vi "Control Panel.vi"(8 "error in (no error)":errorcluster, 11 "Spectrometer iHR320 in":refnum<class "Spectrometer iHR320.lvclass">) -> (0 "error out":errorcluster, 3 "Spectrometer iHR320 out":refnum<class "Spectrometer iHR320.lvclass">)   [LabVIEW 2009, in "Spectrometer iHR320.lvclass"]
doc: "(Dynamic) A user-level application that simulates the physical front panel of the Instrument. Provide the user with buttons to manually control features of the instrument, and provide indicators of its current state."
uses:
  Spectrometer iHR320.lvclass
  Utility Classes/Scannable/Scannable.lvclass
panel:
  in  "Set Filter":bool
  out "Filter Index":i32(ring)=1 items=["Filter 1"=1, "Empty"=2, "Empty"=3, "Empty"=4, "Filter 2"=5, "Filter 3"=6]
  in  "Filter Index Set":i32(ring)=1 items=["Filter 1"=1, "Empty"=2, "Empty"=3, "Empty"=4, "Filter 2"=5, "Filter 3"=6]
  in  "Copy actual to set":bool
  in  "Populate fields with member data":bool
  out "Grating":u16(ring)=1 items=["1200"=1, "600"=2]
  in  "Set Grating":bool
  in  "stop":bool
  in  "Read to control":bool
  in  "Read":bool
  in  "Go To Wavelength":bool
  in  "Set Slit":bool
  in  "Grating set":u16(ring)=1 items=["1200"=1, "600"=2]
  out "Wavelength":dbl[unit]
  in  "Wavelength Set":dbl[unit]
  out "Exit Slit":dbl[unit]
  in  "Exit Slit Set":dbl[unit]
  out "Entrance Slit":dbl[unit]
  in  "Entrance  set":dbl[unit]
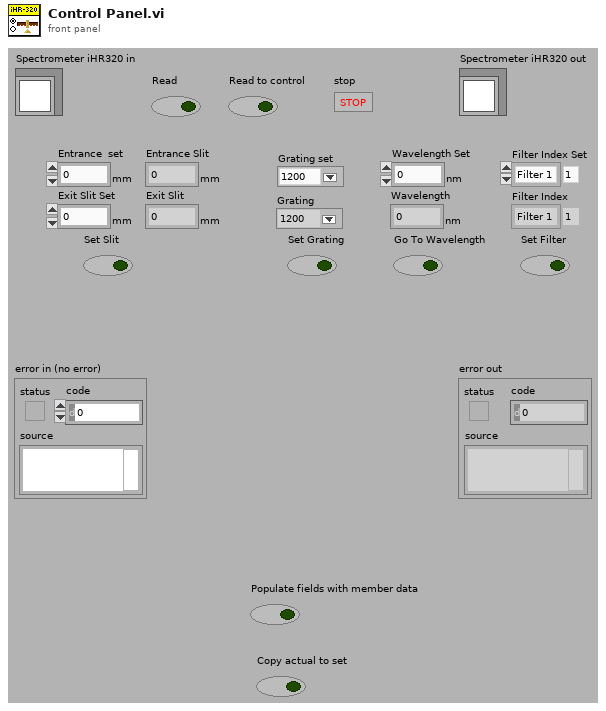
[diagram p1: front panel]
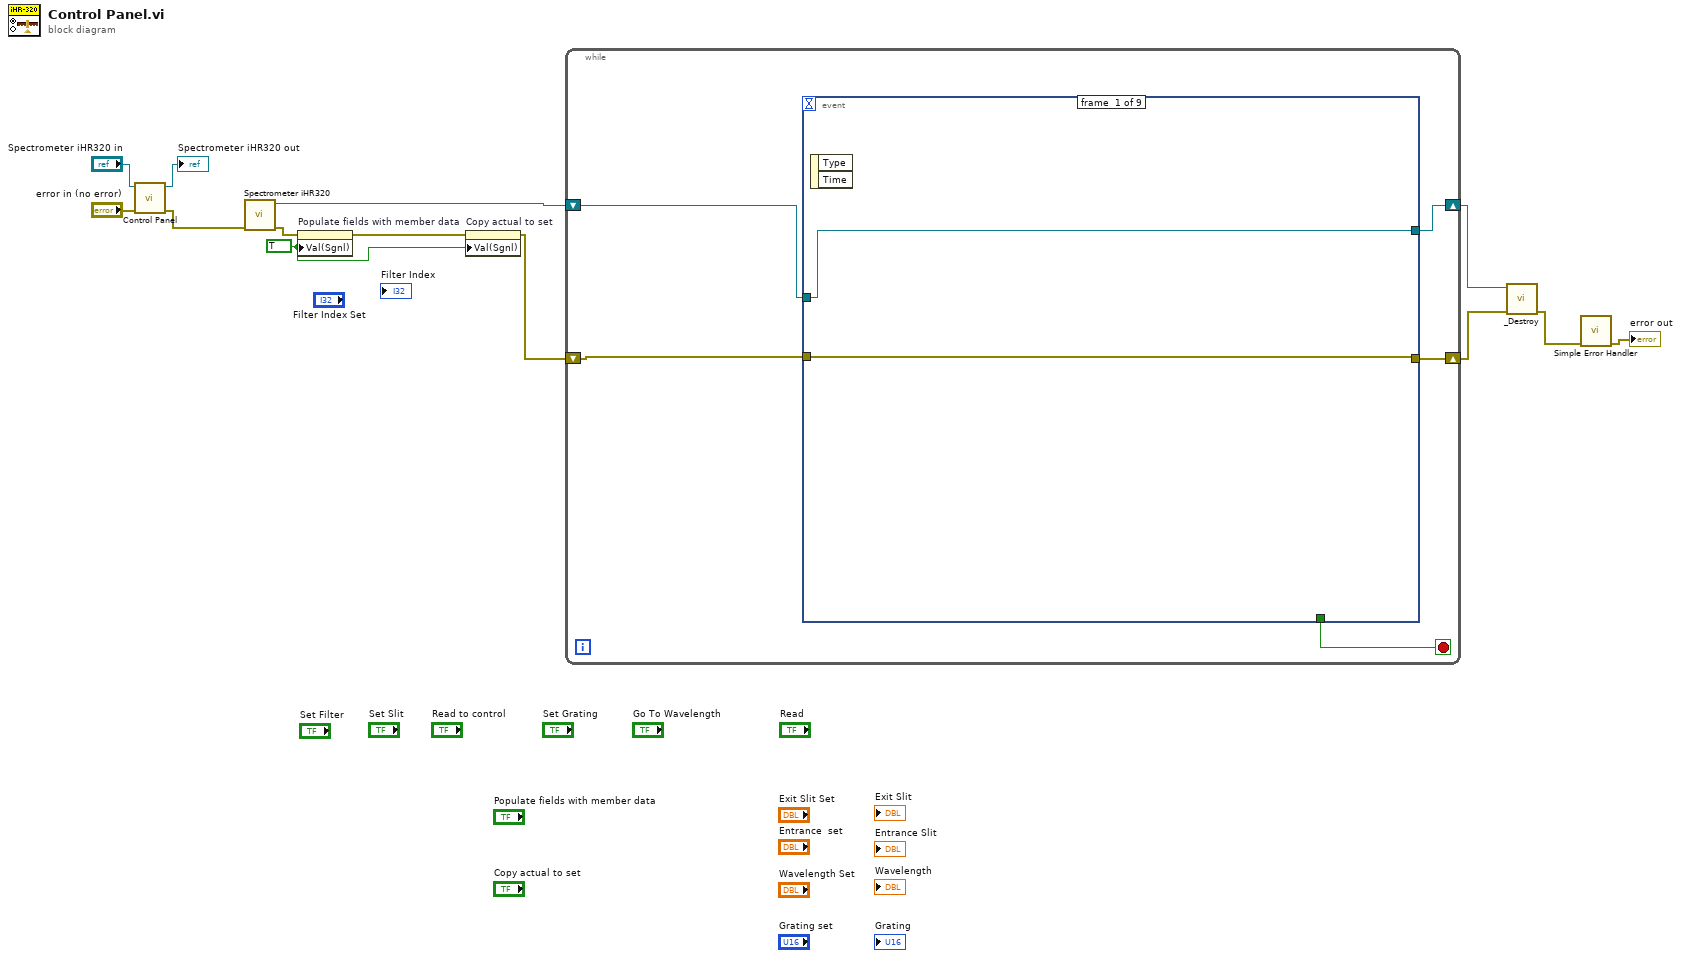
[diagram p0: block diagram]
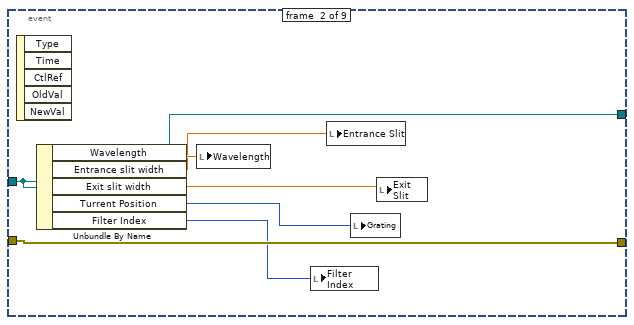
[diagram p2: hidden frame]
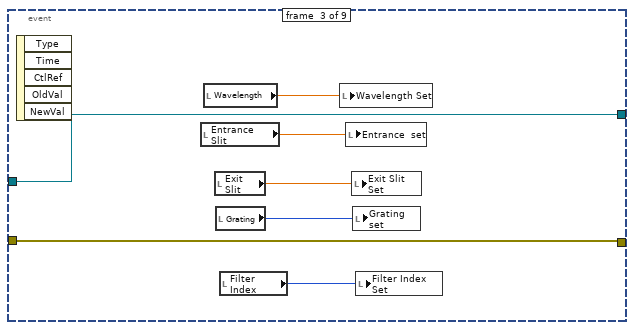
[diagram p3: hidden frame]
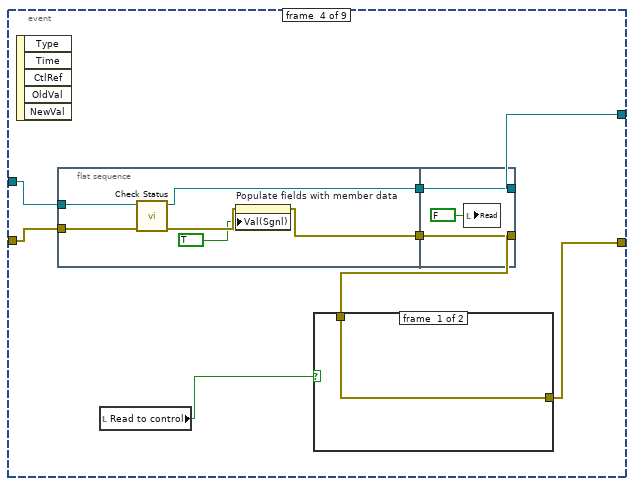
[diagram p4: hidden frame]
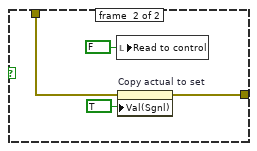
[diagram p5: hidden frame]
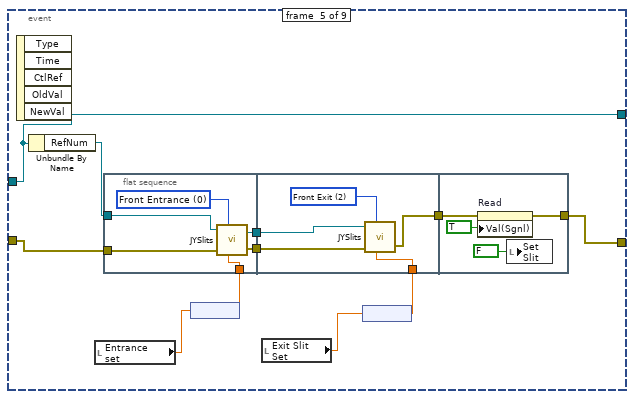
[diagram p6: hidden frame]
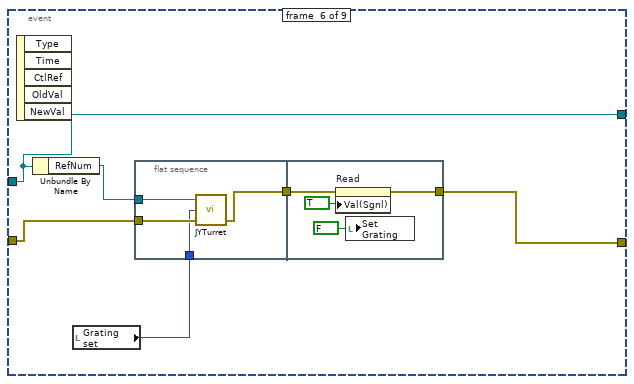
[diagram p7: hidden frame]
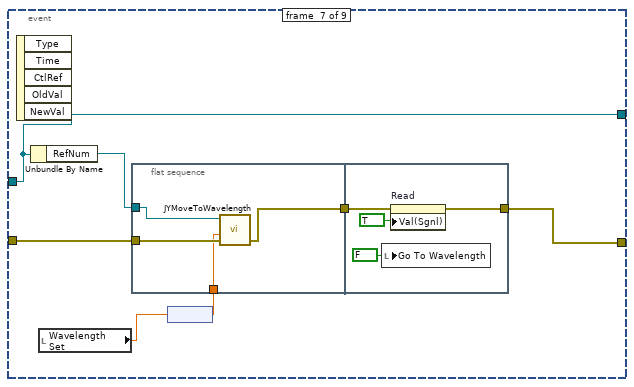
[diagram p8: hidden frame]
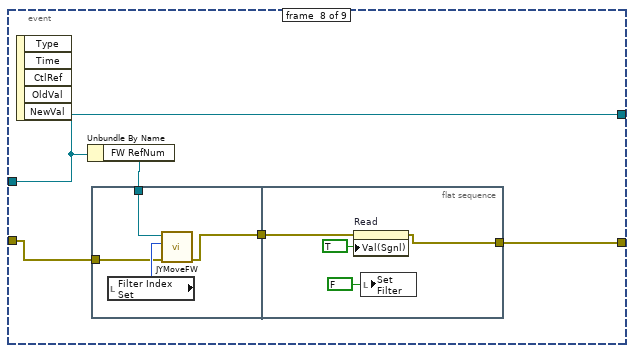
[diagram p9: hidden frame]
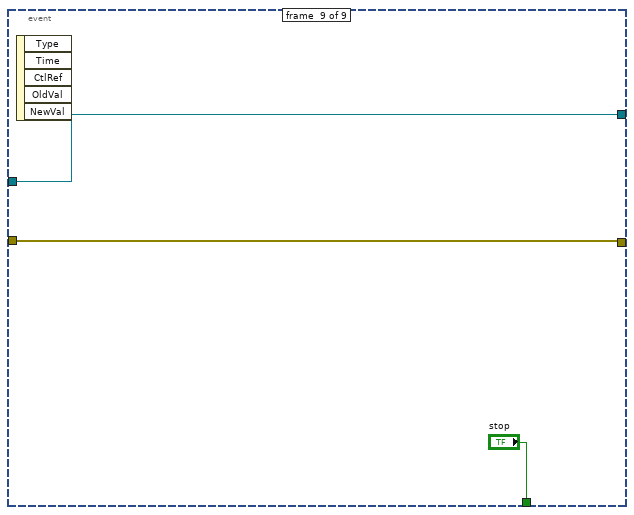
[diagram p10: hidden frame]
diagram:
  w7 = TRUE ("Value (Signaling)")
  n1 = call-parent "Control Panel.vi"("error in (no error)"="error in (no error)", "Instrument in"="Spectrometer iHR320 in") -> ("error out"=w10:errorcluster, "Instrument out"=→"Spectrometer iHR320 out":refnum<class "Spectrometer iHR320.lvclass">)  [unwired: 8 in]
  n2 = call "Spectrometer iHR320.vi"("error in (no error)"=w10) -> ("error out"=w9:errorcluster, "Spectr. iHR320 Out"=w5:refnum<class "Spectrometer iHR320.lvclass">)  [unwired: 9 in]
  n3 = property on="Populate fields with member data" class="Bool (strict)"(error in=w9, "Val(Sgnl)"=w7) -> (error out=w8:errorcluster)  [unwired: 1 in, 1 out]
  n4 = property on="Copy actual to set" class="Bool (strict)"(error in=w8, "Val(Sgnl)"=w7) -> (error out=w6:errorcluster)  [unwired: 1 in, 1 out]
  n5 = while {
    shift-right: [w16] -> w2
    shift-left: w6 -> [w18]
    shift-right: [w15] -> w3
    shift-left: w5 -> [w17]
    stop <- w14 stop-if-true
    n6 = event shown="[2] \"Copy actual to set\": Value Change" {
      selector: _ -> [_ _ _ _ _ _ _ _ _]
      dyn-events: _ -> [_ _ _ _ _ _ _ _ _]
      timeout: _ -> [_ _ _ _ _ _ _ _ _]
      tunnel: w18 -> [w20 w23 w29 w42 w64 w87 w103 w114 w127]
      tunnel: w17 -> [w19 w22 w30 w41 w57 w83 w97 w116 w126]
      tunnel: [w20 w23 w29 w36 w65 w85 w98 w112 w127] -> w16
      tunnel: [w19 w22 w30 w35 w57 w83 w97 w116 w126] -> w15
      tunnel: [_ _ _ _ _ _ _ _ "stop"] -> w14
      event #0 {
        n7 = event-data() -> ()  [unwired: 1 in, 2 out]
      }
      event #1 {
        n8 = event-data() -> ()  [unwired: 1 in, 5 out]
        n9 = Unbundle By Name(w22) -> ("Wavelength"=w27:dbl[unit], "Entrance slit width"=w26:dbl[unit], "Exit slit width"=w25:dbl[unit], "Turrent Position"=w24:u16, "Filter Index"=w21:i32)
        n10 = local write "Wavelength"(w27) -> ()
        n11 = local write "Filter Index"(w21) -> ()
        n12 = local write "Entrance Slit"(w26) -> ()
        n13 = local write "Grating"(w24) -> ()
        n14 = local write "Exit Slit"(w25) -> ()
      }
      event #2 {
        n15 = event-data() -> ()  [unwired: 1 in, 5 out]
        n16 = local read "Entrance Slit"() -> (w33:dbl[unit])
        n17 = local read "Wavelength"() -> (w34:dbl[unit])
        n18 = local read "Exit Slit"() -> (w32:dbl[unit])
        n19 = local read "Grating"() -> (w31:u16)
        n20 = local read "Filter Index"() -> (w28:i32)
        n21 = local write "Wavelength Set"(w34) -> ()
        n22 = local write "Entrance  set"(w33) -> ()
        n23 = local write "Exit Slit Set"(w32) -> ()
        n24 = local write "Grating set"(w31) -> ()
        n25 = local write "Filter Index Set"(w28) -> ()
      }
      event #3 {
        n26 = event-data() -> ()  [unwired: 1 in, 5 out]
        n27 = flat-sequence {
          tunnel: w42 -> [w53]
          tunnel: w41 -> [w52]
          tunnel: [w49] -> w40
          tunnel: [w48] -> w39
          tunnel: [w55] -> w37
          tunnel: w40 -> [w55]
          tunnel: [w54] -> w35
          tunnel: w39 -> [w54]
          frame #0 {
            n28 = call-dynamic "Check Status.vi"("error in (no error)"=w53, "Spectrometer iHR320 in"=w52) -> ("error out"=w51:errorcluster, "Spectrometer iHR320 out"=w48:refnum<class "Spectrometer iHR320.lvclass">)  [unwired: 6 in, 2 out]
            n29 = property on="Populate fields with member data" class="Bool (strict)"(error in=w51, "Val(Sgnl)"=TRUE ("Value (Signaling)")) -> (error out=w49:errorcluster)  [unwired: 1 in, 1 out]
          }
          frame #1 {
            n30 = local write "Read"(FALSE ("Read")) -> ()
          }
        }
        n31 = local read "Read to control"() -> (w38:bool)
        n32 = case shown="False" w38 {
          tunnel: w37 -> [w43 w45]
          tunnel: [w43 w44] -> w36
          frame #0 {
          }
          frame #1 {
            n33 = local write "Read to control"(FALSE ("Read to control")) -> ()
            n34 = property on="Copy actual to set" class="Bool (strict)"(error in=w45, "Val(Sgnl)"=TRUE ("Value (Signaling)")) -> (error out=w44:errorcluster)  [unwired: 1 in, 1 out]
          }
        }
      }
      event #4 {
        n35 = event-data() -> ()  [unwired: 1 in, 5 out]
        n36 = Unbundle By Name(w57) -> ("RefNum"=w63:refnum<k7>)
        n37 = local read "Entrance  set"() -> (w61:dbl[unit])
        n38 = flat-sequence {
          tunnel: [w72] -> w67
          tunnel: w64 -> [w71]
          tunnel: w63 -> [w70]
          tunnel: [w69] -> w62
          tunnel: w60 -> [w68]
          tunnel: w67 -> [w77]
          tunnel: [w76] -> w66
          tunnel: w62 -> [w75]
          tunnel: w58 -> [w74]
          tunnel: w66 -> [w80]
          tunnel: [w79] -> w65
          frame #0 {
            w73 = u16 0 items=["Front Entrance", "Side Entrance", "Front Exit", "Side Exit", "First Intermediate", "Second Intermediate"] ("Slit")
            n39 = call "JYSlits.vi"("JYMONOLib.IJYMonoReqd In"=w70, "Slit"=w73, "error in (no error)"=w71, "Slit Width"=w68) -> ("JYMONOLib.IJYMonoReqd Out"=w69:refnum<k7>, "error out"=w72:errorcluster)  [unwired: 1 in]
          }
          frame #1 {
            w78 = u16 2 items=["Front Entrance", "Side Entrance", "Front Exit", "Side Exit", "First Intermediate", "Second Intermediate"] ("Slit")
            n40 = call "JYSlits.vi"("JYMONOLib.IJYMonoReqd In"=w75, "Slit"=w78, "error in (no error)"=w77, "Slit Width"=w74) -> ("error out"=w76:errorcluster)  [unwired: 1 in, 1 out]
          }
          frame #2 {
            n41 = property on="Read" class="Bool (strict)"(error in=w80, "Val(Sgnl)"=TRUE ("Value (Signaling)")) -> (error out=w79:errorcluster)  [unwired: 1 in, 1 out]
            n42 = local write "Set Slit"(FALSE ("Set Slit")) -> ()
          }
        }
        n43 = node(w61) -> (w60:dbl)
        n44 = local read "Exit Slit Set"() -> (w59:dbl[unit])
        n45 = node(w59) -> (w58:dbl)
      }
      event #5 {
        n46 = event-data() -> ()  [unwired: 1 in, 5 out]
        n47 = Unbundle By Name(w83) -> ("RefNum"=w88:refnum<k7>)
        n48 = local read "Grating set"() -> (w84:u16)
        n49 = flat-sequence {
          tunnel: w88 -> [w92]
          tunnel: w87 -> [w91]
          tunnel: [w90] -> w86
          tunnel: w84 -> [w89]
          tunnel: w86 -> [w94]
          tunnel: [w93] -> w85
          frame #0 {
            n50 = call "JYTurret.vi"("error in (no error)"=w91, "Grating Index"=w89, "JYMONOLib.IJYMonoReqd In"=w92) -> ("error out"=w90:errorcluster)  [unwired: 2 out]
          }
          frame #1 {
            n51 = property on="Read" class="Bool (strict)"(error in=w94, "Val(Sgnl)"=TRUE ("Value (Signaling)")) -> (error out=w93:errorcluster)  [unwired: 1 in, 1 out]
            n52 = local write "Set Grating"(FALSE ("Set Grating")) -> ()
          }
        }
      }
      event #6 {
        n53 = event-data() -> ()  [unwired: 1 in, 5 out]
        n54 = Unbundle By Name(w97) -> ("RefNum"=w101:refnum<k7>)
        n55 = local read "Wavelength Set"() -> (w100:dbl[unit])
        n56 = flat-sequence {
          tunnel: w103 -> [w107]
          tunnel: [w106] -> w102
          tunnel: w101 -> [w105]
          tunnel: w99 -> [w104]
          tunnel: w102 -> [w109]
          tunnel: [w108] -> w98
          frame #0 {
            n57 = call "JYMoveToWavelength.vi"("error in (no error)"=w107, "Target WL"=w104, "RefNum In"=w105) -> ("error out"=w106:errorcluster)  [unwired: 1 in, 2 out]
          }
          frame #1 {
            n58 = local write "Go To Wavelength"(FALSE ("Go To Wavelength")) -> ()
            n59 = property on="Read" class="Bool (strict)"(error in=w109, "Val(Sgnl)"=TRUE ("Value (Signaling)")) -> (error out=w108:errorcluster)  [unwired: 1 in, 1 out]
          }
        }
        n60 = node(w100) -> (w99:dbl)
      }
      event #7 {
        n61 = event-data() -> ()  [unwired: 1 in, 5 out]
        n62 = Unbundle By Name(w116) -> ("FW RefNum"=w115:refnum<k7>)
        n63 = flat-sequence {
          tunnel: w115 -> [w120]
          tunnel: w114 -> [w118]
          tunnel: [w117] -> w113
          tunnel: w113 -> [w122]
          tunnel: [w121] -> w112
          frame #0 {
            n64 = local read "Filter Index Set"() -> (w119:i32)
            n65 = call "JYMoveFW.vi"("error in (no error)"=w118, "Filter Index"=w119, "FW RefNum In"=w120) -> ("error out"=w117:errorcluster)  [unwired: 7 in, 1 out]
          }
          frame #1 {
            n66 = property on="Read" class="Bool (strict)"(error in=w122, "Val(Sgnl)"=TRUE ("Value (Signaling)")) -> (error out=w121:errorcluster)  [unwired: 1 in, 1 out]
            n67 = local write "Set Filter"(FALSE ("Set Filter")) -> ()
          }
        }
      }
      event #8 {
        n68 = event-data() -> ()  [unwired: 1 in, 5 out]
      }
    }
  }
  n69 = call-dynamic "_Destroy.vi"("error in (no error)"=w2, "Spectrometer iHR320 in"=w3) -> ("error out"=w1:errorcluster)  [unwired: 9 in]
  n70 = call <vilib>:"Simple Error Handler.vi"("error in (no error)"=w1) -> ("error out"=→"error out":errorcluster)  [unwired: 4 in, 4 out]
